vi "1_8.vi"() -> ()   [LabVIEW 2020]
panel:
  out "OUT":string
  in  "IN":string
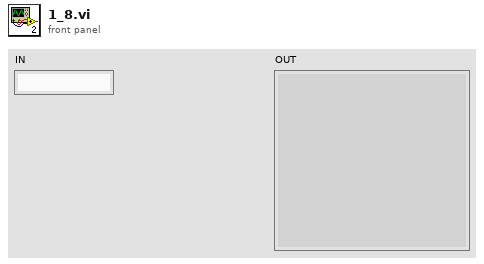
[diagram p1: front panel]
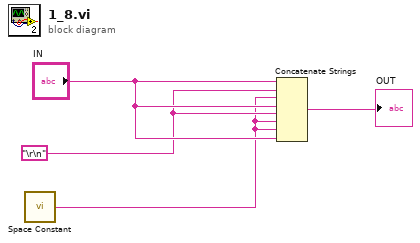
[diagram p0: block diagram]
diagram:
  w2 = "\r\n"
  n1 = call <vilib>:"Space Constant.vi"() -> ("String"=w1:string)
  n2 = Concatenate Strings("IN", w2, w1, "IN", w2, w1, w1, "IN") -> (→"OUT":string)
